vi "APC_9056_ToilControl.vi"(1 "LoadIni?":bool, 2 "PC_ControlSettings":T1={"Spark advance [CADBTDC]"=0.0, "Pref"=0.0, "O2ref"=0.0, "DI advance [CADBTDC]"=0.0, "DI duration [ms] "=0.0, "CO2ref"=0.0, "PFI duration [ms]"=0.0, "IMEP ref"=0.0, "Speed ref"=0.0, "IGN enable"=TRUE, "DI enable"=TRUE, "CL PFI\n lambda"=TRUE, "CL PFI\nIMEP"=FALSE, "Activate\ncylinder"=[FALSE, FALSE, FALSE, FALSE, FALSE, FALSE], "Force idling"=FALSE, "Force motoring"=FALSE, "ETP resync"=FALSE, "Requested mode"=0, "Clear Sync Errors"=FALSE, "toggle TDC"=FALSE, "l ref"=0.0, "PID control references"={"NG"=FALSE, "Ar"=FALSE, "O2"=FALSE, "Intake vent"=FALSE, "Cross vent"=FALSE, "Exhaust vent"=FALSE, "NG control mode"=0, "NG-FC-001-REF"=0.0, "WF-OA-002-REF"=0.0, "IMEP-REF"=0.0, "Nm-REF"=0.0, "Ar control mode"=0, "AR-PC-002-REF"=0.0, "WF-PT-004-REF"=0.0, "O2 control mode"=0, "O2-FC-001-REF"=0.0, "WF-OA-001-REF"=0.0, "Tcoolant control  mode"=0, "EC-FC-001-REF"=0.0, "EC-TT-001-REF"=0.0, "Texh control mode"=0, "SW-FC-004-REF"=0.0, "SW-FT-002-REF"=0.0, "WF-TT-004-REF"=0.0, "Toil control mode"=0, "SW-FC-009-REF"=0.0, "SW-FT-004-REF"=0.0, "EO-TT-001-REF"=0.0, "AIC201_CO2_ConcTarget"=0.0, "O2_FF_NG"=FALSE, "Dyno control mode"=0, "Membrane control mode"=0, "AR-FT-001-REF"=0.0, "MTR modbus floats"=[0.0, 0.0, 0.0, 0.0, 0.0, 0.0, 0.0, 0.0, 0.0, 0.0, 0.0, 0.0, 0.0, 0.0, 0.0, 0.0, 0.0, 0.0, 0.0], "MTR modbus u16"=[0, 0, 0, 0, 0, 0, 0], "MTR HB"=FALSE, "PC_HB"=FALSE, "EMERGENCY STOP"=FALSE}, "CA50setpoint [CADATDC]"=0.0, "CA50 control"=TRUE, "Knock control"=TRUE, "CLEAR EMERGENCY STOP"=FALSE, "EMERGENCY STOP"=FALSE}, 3 "input cluster":T3) -> (0 "SW-FC-009-REF":dbl format="%.2f")   [LabVIEW 2020]
uses:
  controls/APC_PIDCluster.ctl
  controls/APC_ControlSettings.ctl
  controls/APC_PIDcontrolSettings.ctl
  controls/APC_cascadePIDsettings.ctl
  <vilib>/addons/control/pid/pid.llb/PID Advanced (DBL).vi
  <vilib>/Utility/xml.llb/Read From XML File(string).vi
  <vilib>/Utility/xml.llb/Write to XML File(string).vi
  <vilib>/addons/control/pid/NI_PID_pid.lvlib
panel:
  out "direct?":bool
  out "Direct control":dbl format="%.2f"
  in  "SW-FC-009-REF (manual)":dbl
  in  "save":bool
  in  "load":bool
  out "Toil control mode":u8
  out "SW-FT-004":dbl=1.5735627158619593e-07
  in  "LL FF control":dbl format="%.2f"
  in  "reinitialize LL? (F)":bool
  out "EO-TT-001":dbl=2293.706856346882
  in  "SW-FT-004-REF (manual)":dbl
  in  "EO-TT-001-REF (manual)":dbl
  in  "Toil control mode (manual)":u8
  out "HL on?":bool
  out "HL setpoint":dbl format="%.2f"
  in  "LL PID gains":T4={"proportional gain (Kc)"=1.0, "integral time (Ti, min)"=0.01, "derivative time (Td, min)"=0.0} {"derivative time (Td, min)" format="%.3f"; "integral time (Ti, min)" format="%.3f"; "proportional gain (Kc)" format="%.3f"}
  in  "LL PID setpoint range":cluster{"setpoint high":dbl, "setpoint low":dbl}={"setpoint high"=100.0, "setpoint low"=0.0} {"setpoint high" format="%.2f"; "setpoint low" format="%.2f"}
  in  "LL PID output range":cluster{"output high":dbl, "output low":dbl}={"output high"=100.0, "output low"=-100.0} {"output low" format="%.2f"; "output high" format="%.2f"}
  in  "Override PC PID references":bool
  in  "HL learn?":bool
  in  "HL FF control":dbl format="%.2f"
  in  "HL PID gains":T4={"proportional gain (Kc)"=1.0, "integral time (Ti, min)"=0.01, "derivative time (Td, min)"=0.0} {"derivative time (Td, min)" format="%.3f"; "integral time (Ti, min)" format="%.3f"; "proportional gain (Kc)" format="%.3f"}
  in  "HL PID setpoint range":cluster{"setpoint high":dbl, "setpoint low":dbl}={"setpoint high"=100.0, "setpoint low"=0.0} {"setpoint high" format="%.2f"; "setpoint low" format="%.2f"}
  in  "HL PID output range":cluster{"output high":dbl, "output low":dbl}={"output high"=100.0, "output low"=-100.0} {"output low" format="%.2f"; "output high" format="%.2f"}
  in  "Safe mode control":dbl format="%.2f"
  in  "LL learn?":bool
  in  "reinitialize HL? (F)":bool
  out "LL on?":bool
  out "LL setpoint":dbl format="%.2f"
  # "Toil control"
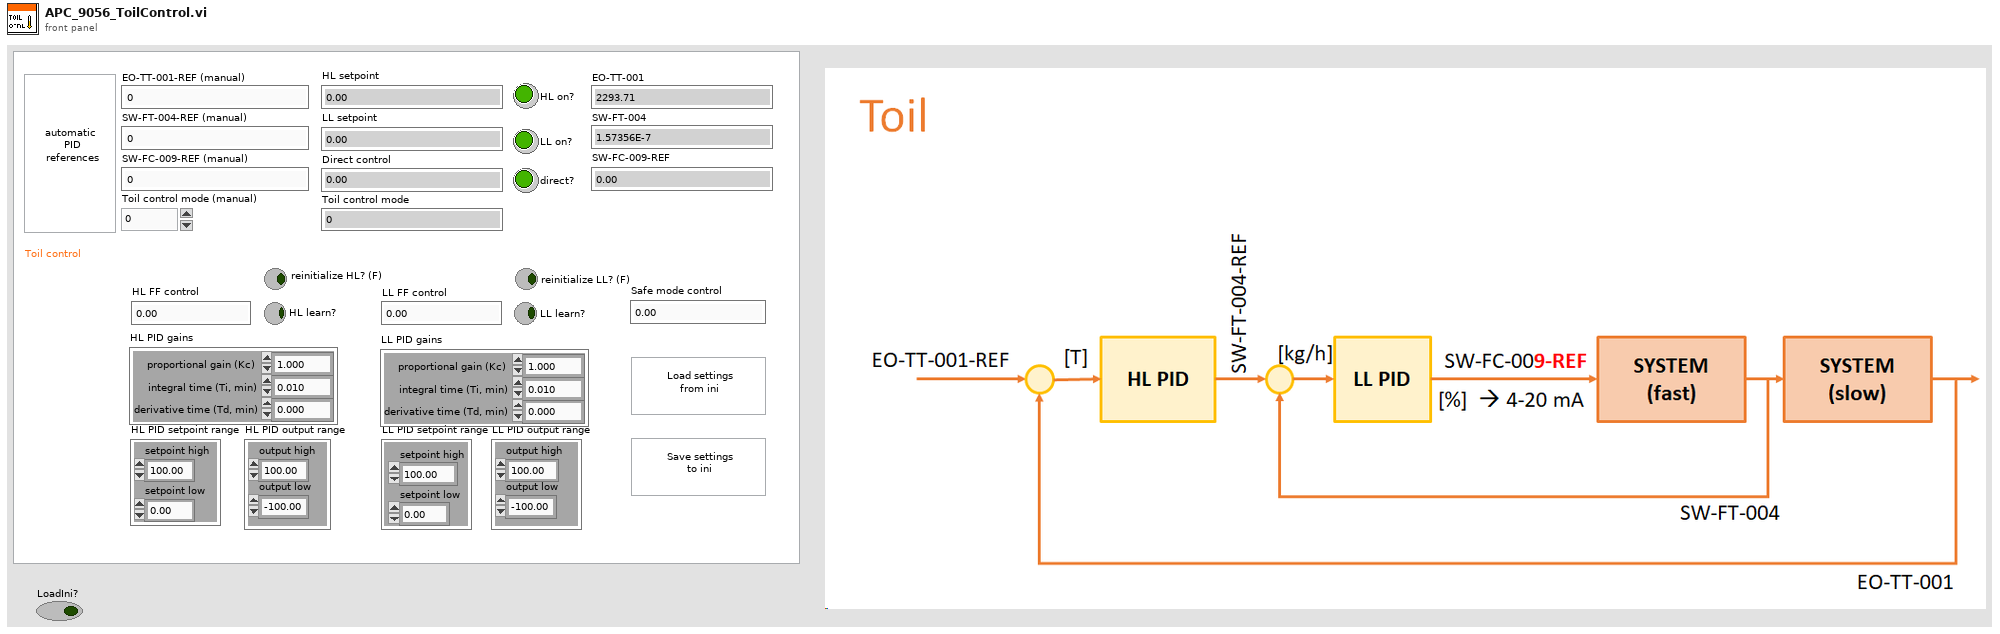
[diagram p1: front panel]
types:
  T1 = typedef "APC_ControlSettings.ctl" = cluster{"Spark advance [CADBTDC]":dbl, "Pref":dbl, "O2ref":dbl, "DI advance [CADBTDC]":dbl, "DI duration [ms] ":dbl, "CO2ref":dbl, "PFI duration [ms]":dbl, "IMEP ref":dbl, "Speed ref":dbl, "IGN enable":bool, "DI enable":bool, "CL PFI\n lambda":bool, "CL PFI\nIMEP":bool, "Activate\ncylinder":bool[], "Force idling":bool, "Force motoring":bool, "ETP resync":bool, "Requested mode":i8, "Clear Sync Errors":bool, "toggle TDC":bool, "l ref":dbl, "PID control references":T2, "CA50setpoint [CADATDC]":dbl, "CA50 control":bool, "Knock control":bool, "CLEAR EMERGENCY STOP":bool, "EMERGENCY STOP":bool}
  T2 = typedef "APC_PIDcontrolSettings.ctl" = cluster{"NG":bool, "Ar":bool, "O2":bool, "Intake vent":bool, "Cross vent":bool, "Exhaust vent":bool, "NG control mode":u8, "NG-FC-001-REF":dbl, "WF-OA-002-REF":dbl, "IMEP-REF":dbl, "Nm-REF":dbl, "Ar control mode":u8, "AR-PC-002-REF":dbl, "WF-PT-004-REF":dbl, "O2 control mode":u8, "O2-FC-001-REF":dbl, "WF-OA-001-REF":dbl, "Tcoolant control  mode":u8, "EC-FC-001-REF":dbl, "EC-TT-001-REF":dbl, "Texh control mode":u8, "SW-FC-004-REF":dbl, "SW-FT-002-REF":dbl, "WF-TT-004-REF":dbl, "Toil control mode":u8, "SW-FC-009-REF":dbl, "SW-FT-004-REF":dbl, "EO-TT-001-REF":dbl, "AIC201_CO2_ConcTarget":dbl, "O2_FF_NG":bool, "Dyno control mode":u8, "Membrane control mode":u8, "AR-FT-001-REF":dbl, "MTR modbus floats":sgl[], "MTR modbus u16":u16[], "MTR HB":bool, "PC_HB":bool, "EMERGENCY STOP":bool}
  T3 = typedef "APC_PIDCluster.ctl" = cluster{"AR-FT-001":dbl, "O2-FC-001":dbl, "SW-FT-004":dbl, "SW-FT-002":dbl, "WF-OA-002":dbl, "WF-PT-004":dbl, "WF-OA-001":dbl, "EC-TT-001":dbl, "WF-TT-004":dbl, "EC-FC-001":dbl, "NG-FC-001":dbl, "EO-TT-001":dbl, "SW-FC-008":dbl, "SW-FC-004":dbl, "IMEPn6":dbl, "TORQUE":dbl, "CylPresWarnings":dbl, "CylPresErrors":dbl, "NG-FT-001":dbl, "EngineSpeed_rpm":dbl}
  T4 = cluster{"proportional gain (Kc)":dbl, "integral time (Ti, min)":dbl, "derivative time (Td, min)":dbl}
  T5 = typedef "APC_cascadePIDsettings.ctl" = cluster{"HL FF control":dbl, "LL FF control":dbl, "HL PID gains":cluster{"proportional gain (Kc)":dbl, "integral time (Ti, min)":dbl, "derivative time (Td, min)":dbl}, "LL PID gains":cluster{"proportional gain (Kc)":dbl, "integral time (Ti, min)":dbl, "derivative time (Td, min)":dbl}, "HL PID setpoint range":cluster{"setpoint high":dbl, "setpoint low":dbl}, "HL PID output range":cluster{"output high":dbl, "output low":dbl}, "LL PID setpoint range":cluster{"setpoint high":dbl, "setpoint low":dbl}, "LL PID output range":cluster{"output high":dbl, "output low":dbl}, "Safe mode control":dbl}
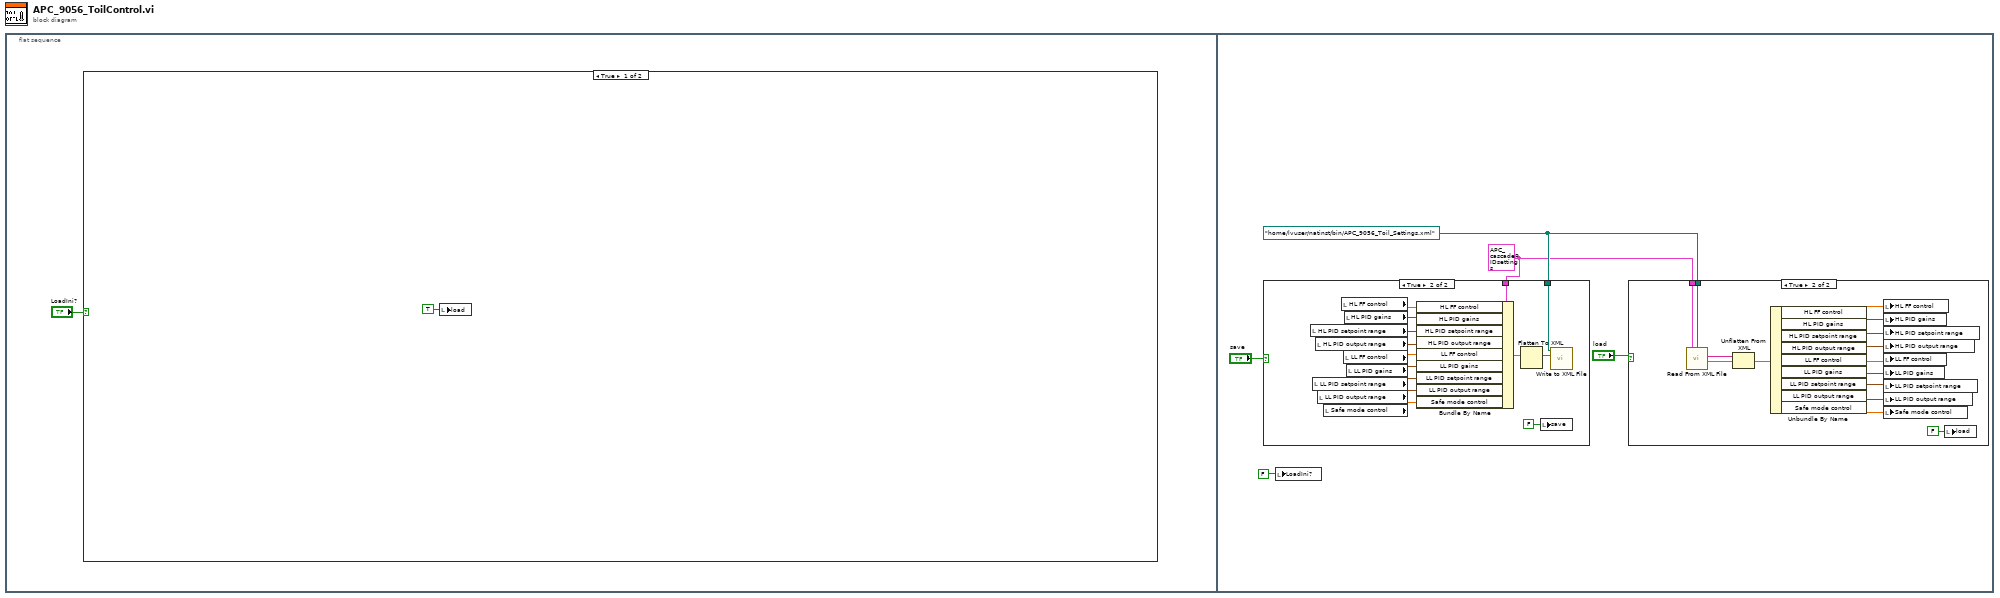
[diagram p0: block diagram]
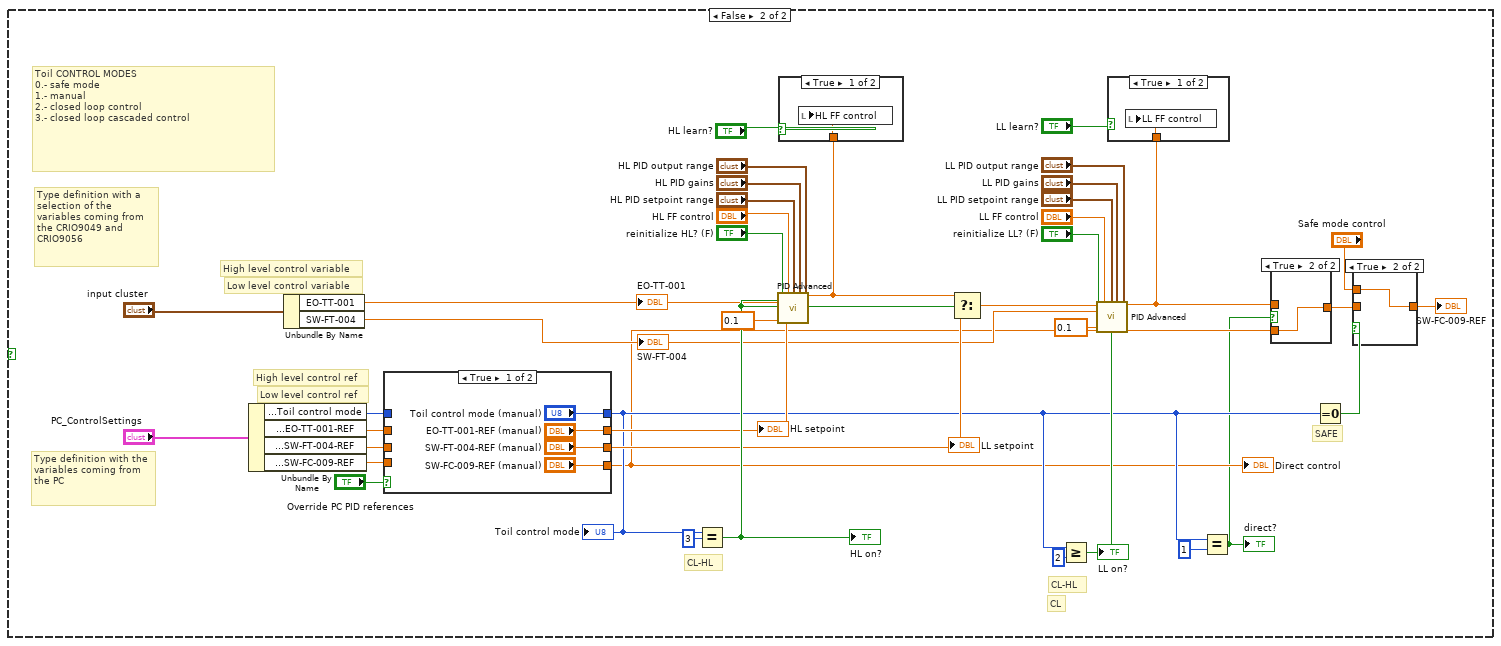
[diagram p2: hidden frame]
diagram:
  n1 = flat-sequence {
    frame #0 {
      n2 = case shown="True" "LoadIni?" {
        frame True {
          n3 = local write "load"(TRUE ("load")) -> ()
        }
        frame False {
          # "Type definition with a selection of the variables coming from the CRIO9049 and CRIO9056"
          # "Type definition with the variables coming from the PC"
          # "CL-HL"
          # "Low level control ref"
          # "Low level control variable"
          # "High level control ref"
          # "High level control variable"
          # "SAFE"
          # "CL-HL"
          # "CL"
          # "Toil CONTROL MODES\n0.- safe mode\n1.- manual\n2.- closed loop control \n3.- closed loop cascaded control"
          n4 = Unbundle By Name("PC_ControlSettings") -> ("PID control references.Toil control mode"=w19:u8, "PID control references.EO-TT-001-REF"=w18:dbl, "PID control references.SW-FT-004-REF"=w17:dbl, "PID control references.SW-FC-009-REF"=w9:dbl)
          n5 = Unbundle By Name("input cluster") -> ("EO-TT-001"=w16:dbl, "SW-FT-004"=w12:dbl)
          "EO-TT-001" <- w16
          "SW-FT-004" <- w12
          n6 = case shown="True" "Override PC PID references" {
            tunnel: w19 -> [_ w56]
            tunnel: w18 -> [_ w55]
            tunnel: w17 -> [_ w54]
            tunnel: ["Toil control mode (manual)" w56] -> w8
            tunnel: ["EO-TT-001-REF (manual)" w55] -> w15
            tunnel: ["SW-FT-004-REF (manual)" w54] -> w14
            tunnel: w9 -> [_ w53]
            tunnel: ["SW-FC-009-REF (manual)" w53] -> w4
            frame True {
            }
            frame False {
            }
          }
          "LL setpoint" <- w14
          "HL setpoint" <- w15
          "Toil control mode" <- w8
          "Direct control" <- w4
          n7 = Equal?(x=w8, y=u8 3) -> (x = y?=w26:bool)
          "HL on?" <- w26
          n8 = call-poly <vilib>:"PID Advanced.vi"("setpoint"=w15, "output range"="HL PID output range", "auto? (T)"=w26, "manual control"="HL FF control", "process variable"=w16, "setpoint range"="HL PID setpoint range", "PID gains"="HL PID gains", "dt (s)"=0.1, "reinitialize? (F)"="reinitialize HL? (F)") -> ("output"=w31:dbl)  [unwired: 5 in, 1 out]
          n9 = case shown="True" "HL learn?" {
            tunnel: w31 -> [w48 _]
            frame True {
              n10 = local write "HL FF control"(w48) -> ()
            }
            frame False {
            }
          }
          n11 = Select(t=w31, s=w26, f=w14) -> (s? t:f=w37:dbl)
          n12 = Greater Or Equal?(x=w8, y=u8 2) -> (x >= y?=w40:bool)
          "LL on?" <- w40
          n13 = call-poly <vilib>:"PID Advanced.vi"("setpoint"=w37, "output range"="LL PID output range", "auto? (T)"=w40, "manual control"="LL FF control", "process variable"=w12, "setpoint range"="LL PID setpoint range", "PID gains"="LL PID gains", "dt (s)"=0.1, "reinitialize? (F)"="reinitialize LL? (F)") -> ("output"=w6:dbl)  [unwired: 5 in, 1 out]
          n14 = case shown="True" "LL learn?" {
            tunnel: w6 -> [w45 _]
            frame True {
              n15 = local write "LL FF control"(w45) -> ()
            }
            frame False {
            }
          }
          n16 = Equal?(x=w8, y=u8 1) -> (x = y?=w3:bool)
          "direct?" <- w3
          n17 = case shown="True" w3 {
            tunnel: [w43 w44] -> w5
            tunnel: w6 -> [w43 _]
            tunnel: w4 -> [_ w44]
            frame False {
            }
            frame True {
            }
          }
          n18 = Equal To 0?(x=w8) -> (x = 0?=w42:bool)
          n19 = case shown="True" w42 {
            tunnel: [w46 w47] -> w25
            tunnel: "Safe mode control" -> [_ w47]
            tunnel: w5 -> [w46 _]
            frame False {
            }
            frame True {
            }
          }
          "SW-FC-009-REF" <- w25
        }
      }
    }
    frame #1 {
      w59 = path "/home/lvuser/natinst/bin/APC_9056_Toil_Settings.xml" ("XML File Path")
      w58 = T5 {"HL FF control"=0.0, "LL FF control"=0.0, "HL PID gains"={"proportional gain (Kc)"=1.0, "integral time (Ti, min)"=0.01, "derivative time (Td, min)"=0.0}, "LL PID gains"={"proportional gain (Kc)"=1.0, "integral time (Ti, min)"=0.01, "derivative time (Td, min)"=0.0}, "HL PID setpoint range"={"setpoint high"=100.0, "setpoint low"=0.0}, "HL PID output range"={"output high"=0.0, "output low"=0.0}, "LL PID setpoint range"={"setpoint high"=100.0, "setpoint low"=0.0}, "LL PID output range"={"output high"=10.0, "output low"=-10.0}, "Safe mode control"=0.0} ("Cluster")
      n20 = case shown="True" "save" {
        tunnel: w59 -> [_ w78]
        tunnel: w58 -> [_ w77]
        frame False {
        }
        frame True {
          n21 = local read "HL PID setpoint range"() -> (w87:cluster{"setpoint high":dbl, "setpoint low":dbl})
          n22 = local read "LL PID setpoint range"() -> (w83:cluster{"setpoint high":dbl, "setpoint low":dbl})
          n23 = local read "HL PID output range"() -> (w86:cluster{"output high":dbl, "output low":dbl})
          n24 = local read "LL PID output range"() -> (w82:cluster{"output high":dbl, "output low":dbl})
          n25 = local read "Safe mode control"() -> (w81:dbl)
          n26 = local read "HL FF control"() -> (w89:dbl)
          n27 = local read "LL FF control"() -> (w85:dbl)
          n28 = local read "HL PID gains"() -> (w88:T4)
          n29 = local read "LL PID gains"() -> (w84:T4)
          n30 = Bundle By Name(cluster=w77, "HL FF control"=w89, "HL PID gains"=w88, "HL PID setpoint range"=w87, "HL PID output range"=w86, "LL FF control"=w85, "LL PID gains"=w84, "LL PID setpoint range"=w83, "LL PID output range"=w82, "Safe mode control"=w81) -> (w80:T5)
          n31 = Flatten To XML(6:w80) -> (2:w79:string)
          n32 = local write "save"(FALSE ("load")) -> ()
          n33 = call-poly <vilib>:"Write to XML File.vi"("XML Input"=w79, "XML File Path"=w78) -> ()  [unwired: 7 in, 3 out]
        }
      }
      n34 = local write "LoadIni?"(FALSE ("LoadIni?")) -> ()
      n35 = case shown="True" "load" {
        tunnel: w59 -> [_ w74]
        tunnel: w58 -> [_ w73]
        frame False {
        }
        frame True {
          n36 = call-poly <vilib>:"Read From XML File.vi"("XML File Path"=w74) -> ("XML Elements"=w75:string)  [unwired: 8 in, 2 out]
          n37 = Unflatten From XML(xml string=w75, type=w73) -> (value=w72:T5)  [unwired: 1 in, 1 out]
          n38 = Unbundle By Name(w72) -> ("HL FF control"=w71:dbl, "HL PID gains"=w70:T4, "HL PID setpoint range"=w69:cluster{"setpoint high":dbl, "setpoint low":dbl}, "HL PID output range"=w68:cluster{"output high":dbl, "output low":dbl}, "LL FF control"=w67:dbl, "LL PID gains"=w66:T4, "LL PID setpoint range"=w65:cluster{"setpoint high":dbl, "setpoint low":dbl}, "LL PID output range"=w64:cluster{"output high":dbl, "output low":dbl}, "Safe mode control"=w63:dbl)
          n39 = local write "HL FF control"(w71) -> ()
          n40 = local write "HL PID gains"(w70) -> ()
          n41 = local write "HL PID setpoint range"(w69) -> ()
          n42 = local write "HL PID output range"(w68) -> ()
          n43 = local write "LL FF control"(w67) -> ()
          n44 = local write "LL PID gains"(w66) -> ()
          n45 = local write "LL PID setpoint range"(w65) -> ()
          n46 = local write "LL PID output range"(w64) -> ()
          n47 = local write "Safe mode control"(w63) -> ()
          n48 = local write "load"(FALSE ("save")) -> ()
        }
      }
    }
  }
